vi "Toggle Display Help.vi"(11 "Scene in":refnum<class "Scene.lvclass">) -> (3 "Scene out":refnum<class "Scene.lvclass">)   [LabVIEW 2020, in "Scene.lvclass"]
uses:
  Scene.lvclass
  Scene.lvclass/Scene.ctl
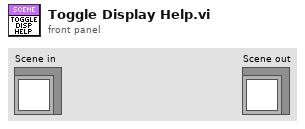
[diagram p1: front panel]
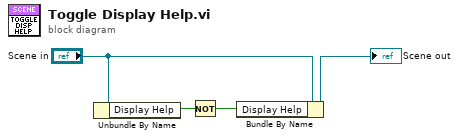
[diagram p0: block diagram]
diagram:
  n1 = Unbundle By Name("Scene in") -> ("Display Help"=w2:bool)
  n2 = Not(x=w2) -> (.not. x?=w1:bool)
  n3 = Bundle By Name(cluster="Scene in", "Display Help"=w1) -> (→"Scene out":refnum<class "Scene.lvclass">)
